vi "splitter Adjust for traverse.vi"(8 "error in":errorcluster caption="错误输入（无错误）", 11 "Class in":refnum<class "PanelRootNode.lvclass"> caption="DNL_LabVIEW Object in") -> (0 "error out":errorcluster caption="错误输出", 3 "Class out":refnum<class "PanelRootNode.lvclass"> caption="DNL_LabVIEW Object out")   [LabVIEW 2013, in "PanelRootNode.lvclass"]
uses:
  PanelRootNode.lvclass
  PanelLinkNode/PanelLinkNode.lvclass/PanelLinkNode.ctl
  PanelObject/PanelObject.lvclass
  PanelLinkNode/PanelLinkNode.lvclass
  PanelDataNode/PanelDataNode.lvclass
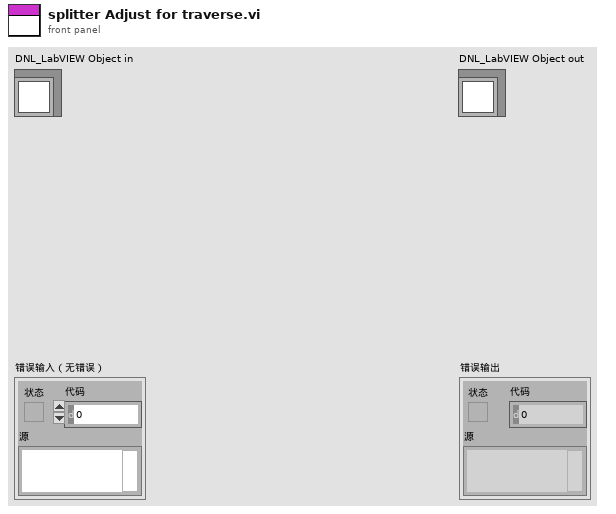
[diagram p1: front panel]
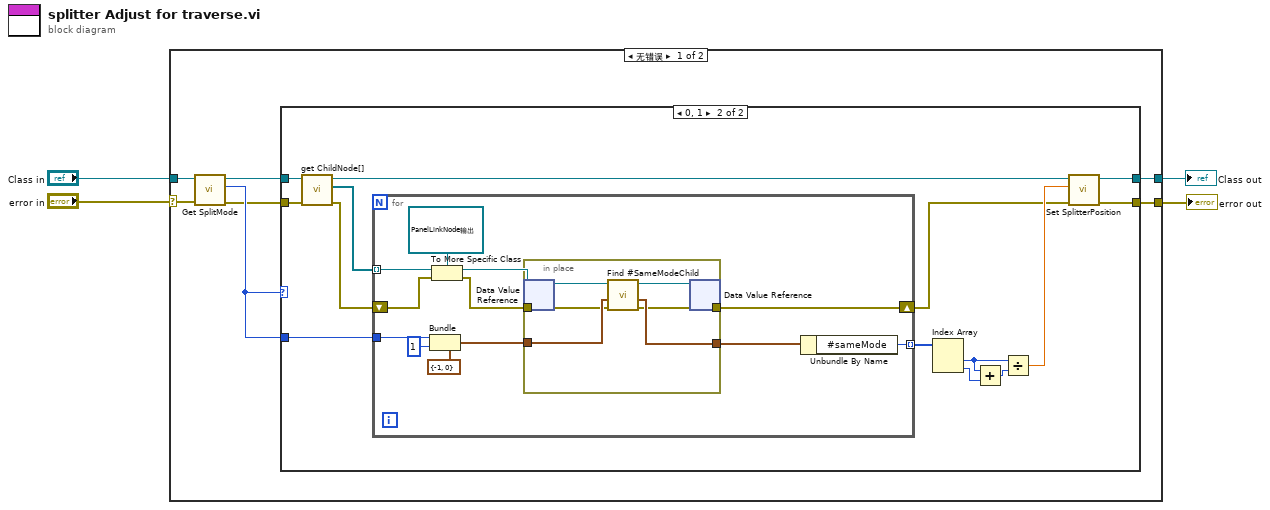
[diagram p0: block diagram]
diagram:
  n1 = case shown="无错误" "error in" {
    selector: "error in" -> [w5 w47]
    tunnel: [w6 w47] -> w3
    tunnel: [w9 w46] -> w1
    tunnel: "Class in" -> [w11 w46]
    frame No Error {
      n2 = call-dynamic "Get SplitMode.vi"("error in (no error)"=w5, "PanelDataNode 输入"=w11) -> ("error out"=w7:errorcluster, "Split Mode"=w8:i32, "PanelDataNode 输出"=w10:refnum<class "PanelRootNode.lvclass">)  [unwired: 7 in]
      n3 = case shown="0, 1" w8 {
        tunnel: w10 -> [w13 w27]
        tunnel: w8 -> [_ w26]
        tunnel: [w13 w22] -> w9
        tunnel: w7 -> [w12 w17]
        tunnel: [w12 w14] -> w6
        frame -1, Default {
        }
        frame 0, 1 {
          n4 = call "get ChildNode[].vi"("error in (no error)"=w17, "PanelLinkNode输入"=w27) -> ("error out"=w16:errorcluster, "ChildNode*[]"=w25:refnum<data-value>[], "PanelLinkNode输出"=w23:refnum<class "PanelRootNode.lvclass">)  [unwired: 7 in]
          n5 = for {
            tunnel: w26 -> [w39]
            tunnel: w25 -> [w35] mode=indexing
            tunnel: [w32] -> w24 mode=indexing
            shift-right: [w30] -> w15
            shift-left: w16 -> [w31]
            n6 = Bundle(cluster=cluster{"Split Mode":i32, "#sameMode":i32} {"Split Mode"=-1, "#sameMode"=0} ("Data in"), "Split Mode"=w39, "#sameMode"=1) -> (w37:cluster{"Split Mode":i32, "#sameMode":i32})
            n7 = To More Specific Class(target class=refnum<data-value> refnum ("数据值引用"), reference=w35, error in=w31) -> (specific class reference=w33:refnum<data-value>, error out=w28:errorcluster)
            n8 = in-place {
              in-place-border: w37 -> [w43]
              in-place-border: [w42] -> w29
              in-place-border: w28 -> [w41]
              in-place-border: [w40] -> w30
              n9 = in-place-dvr #1(w33) -> (w45:refnum<class "PanelRootNode.lvclass">)  [unwired: 1 out]
              n10 = call "Find #SameModeChild.vi"("error in"=w41, "Data in"=w43, "PanelRootNode.lvclass"=w45) -> ("error out"=w40:errorcluster, "Data out"=w42:cluster{"Split Mode":i32, "#sameMode":i32}, "PanelRootNode.lvclass 2"=w44:refnum<class "PanelRootNode.lvclass">)  [unwired: 6 in]
              n11 = in-place-dvr #1(w44) -> ()  [unwired: 2 out]
            }
            n12 = Unbundle By Name(w29) -> ("#sameMode"=w32:i32)
          }
          n13 = Index Array(array=w24) -> (element #1=w21:i32, element #2=w20:i32)  [unwired: 2 in]
          n14 = Add(x=w21, y=w20) -> (x+y=w19:i32)
          n15 = Divide(x=w21, y=w19) -> (x/y=w18:dbl)
          n16 = call "Set SplitterPosition.vi"("error in (no error)"=w15, "Position(relative)"=w18, "PanelDataNode 输入"=w23) -> ("error out"=w14:errorcluster, "PanelDataNode 输出"=w22:refnum<class "PanelRootNode.lvclass">)  [unwired: 7 in]
        }
      }
    }
    frame Error {
    }
  }
  "error out" <- w3
  "Class out" <- w1
